vi "Commit NVMEM for Session.vi"(0 "session in":refnum<k21>, 11 "error in (no error)":errorcluster) -> (4 "session out":refnum<k21>, 15 "error out":errorcluster)   [LabVIEW 2020, in "SLSC.lvlib"]
doc: "Commits pending changes to hardware for all NVMEM areas for all modules in the session. If the session has any chassis reserved, this VI/function skips over them. If you set the same address multiple times between commits, only the last value will be committed."
uses:
  <vilib>/SLSC/SLSC.lvlib
  nislsclvapi.dll
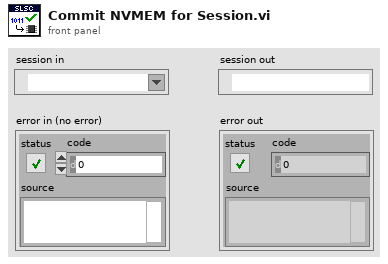
[diagram p1: front panel]
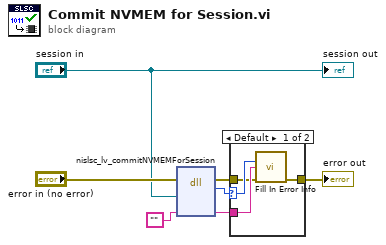
[diagram p0: block diagram]
diagram:
  n1 = dll-call lib="nislsclvapi.*" fn="nislsc_lv_commitNVMEMForSession"(error in="error in (no error)", "session"="session in", "extendedErrorInfo"="") -> (error out=w2:errorcluster, "return type"=w3:i32, "extendedErrorInfo"=w4:string)  [unwired: 5 in, 1 out]
  n2 = case shown="Default" w3 {
    selector: w3 -> [w11 _]
    tunnel: w4 -> [w10 _]
    tunnel: w2 -> [w9 w12]
    tunnel: [w8 w12] -> w1
    frame Default {
      n3 = call <vilib>:"Fill In Error Info.vi"("status code"=w11, "extended error info"=w10, "error in"=w9) -> ("error out"=w8:errorcluster)  [unwired: 12 in]
    }
    frame 0 {
    }
  }
  "error out" <- w1
  "session out" <- "session in"
